vi "Degub.vi"   [LabVIEW 2020]
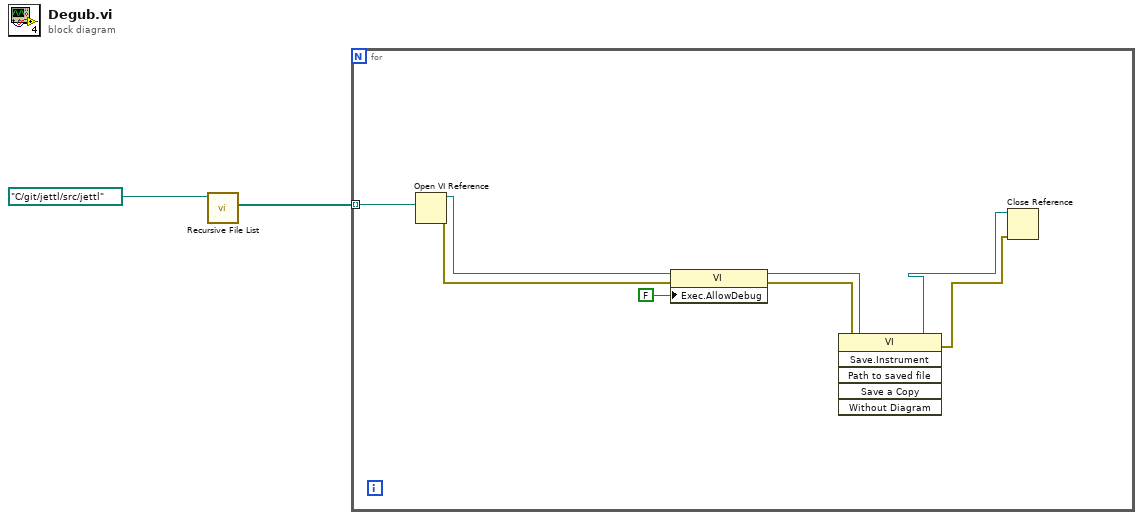
[diagram p0: block diagram]
diagram:
  n1 = call <vilib>:"Recursive File List.vi"("Folder Path"=path "C:/git/jettl/src/jettl" ("Path")) -> ("All Files in Dir"=w2:path[])  [unwired: 6 in, 4 out]
  n2 = for {
    tunnel: w2 -> [w10] mode=indexing
    n3 = Open VI Reference(vi path=w10) -> (vi reference=w8:refnum<vi>, error out=w9:errorcluster)  [unwired: 5 in]
    n4 = property class="VI"(reference=w8, error in=w9, "Exec.AllowDebug"=FALSE ("Execution:Allow Debugging")) -> (reference out=w7:refnum<vi>, error out=w5:errorcluster)
    n5 = invoke class="VI" method="Save.Instrument"(reference=w7, error in=w5) -> (reference out=w6:refnum<vi>, error out=w4:errorcluster)  [unwired: 4 in, 4 out]
    n6 = Close Reference(reference=w6, error in (no error)=w4) -> ()  [unwired: 1 out]
  }
